vi "Simple Add.vi"(9 "Number 3":dbl, 10 "Number 2":dbl, 11 "Number 1":dbl) -> (3 "Result":dbl)   [LabVIEW 2018]
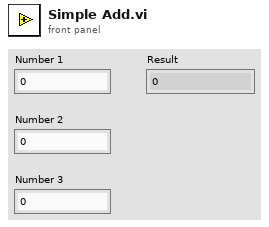
[diagram p1: front panel]
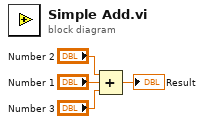
[diagram p0: block diagram]
diagram:
  n1 = Compound Arithmetic op=ADD("Number 2", "Number 1", "Number 3") -> (→"Result":dbl)
